vi "Get_OSC_DS1104Z.vi"(9 "Timeout (10000 ms)":u32=10000, 10 "Channel (0: Channel 1)":u16(ring) items=["Channel 1", "Channel 2", "Channel 3", "Channel 4"], 11 "VISA resource name":refnum<visa-resource-name>) -> (3 "Waveform Data":waveform(dbl)(graph))   [LabVIEW 2018]
panel:
  in  "t":i16=-25
  out "VISA resource name out":refnum<visa-resource-name>
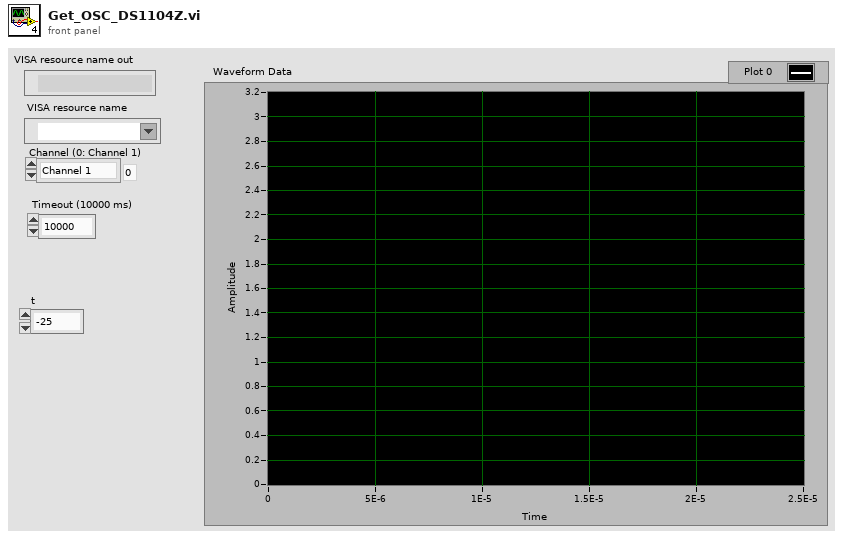
[diagram p1: front panel]
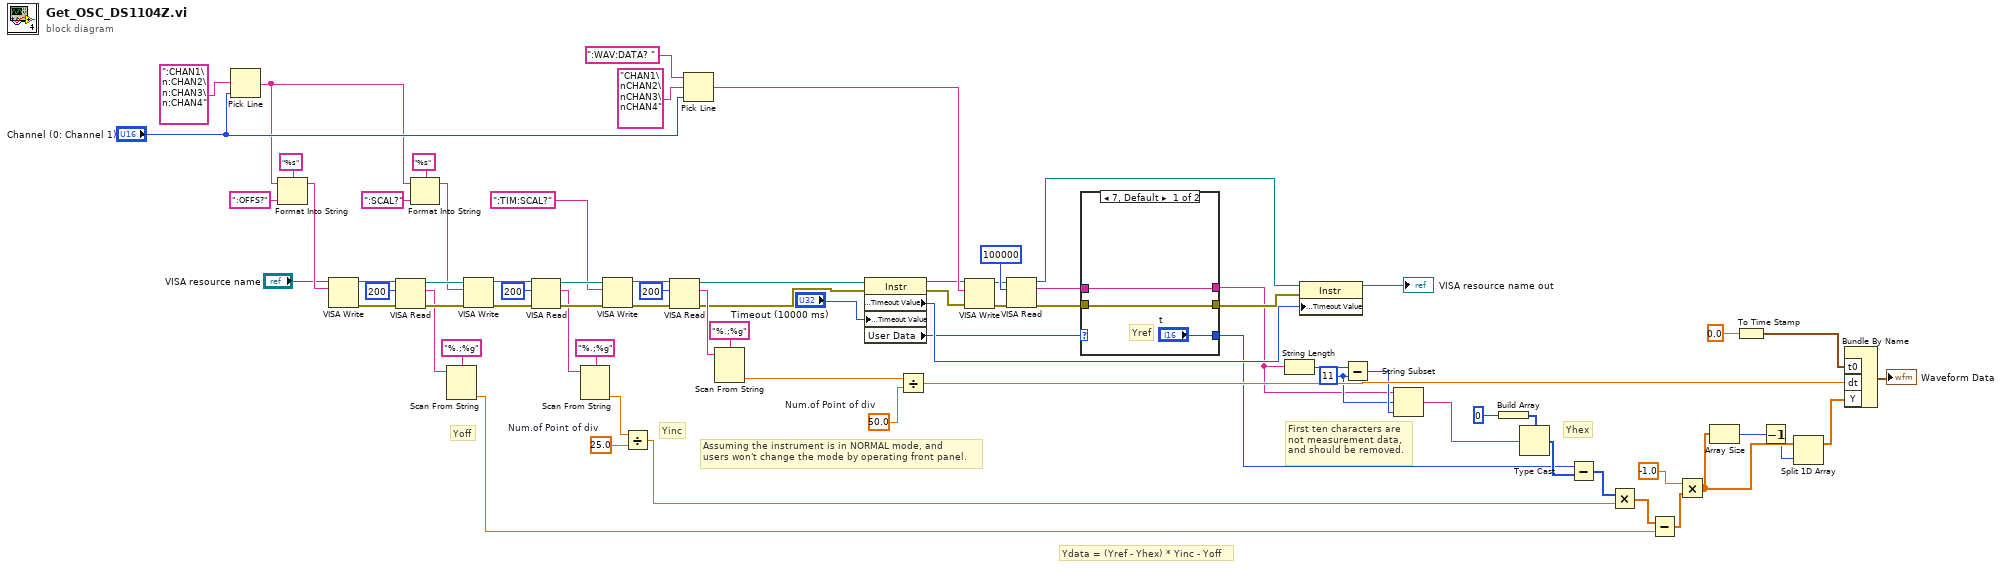
[diagram p0: block diagram]
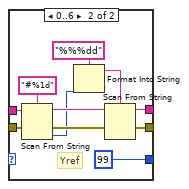
[diagram p2: hidden frame]
diagram:
  w14 = 11 ("y")
  w24 = 50.0  # Num.of Point of div
  w31 = 25.0  # Num.of Point of div
  # "Assuming the instrument is in NORMAL mode, and \nusers won't change the mode by operating front panel."
  # "First ten characters are\nnot measurement data, \nand should be removed."
  # "Yoff"
  # "Yinc"
  # "Yhex"
  # "Ydata = (Yref - Yhex) * Yinc - Yoff"
  n1 = Pick Line(multi-line string=":CHAN1\n:CHAN2\n:CHAN3\n:CHAN4" ("多行字符串"), line index="Channel (0: Channel 1)") -> (output string=w40:string)  [unwired: 1 out]
  n2 = Format Into String(format string="%s" ("格式字符串"), initial string=w40, ":OFFS?") -> (resulting string=w37:string)  [unwired: 1 in, 1 out]
  n3 = VISA Write(VISA resource name="VISA resource name", write buffer=w37) -> (VISA resource name out=w56:refnum<visa-resource-name>, error out=w55:errorcluster)  [unwired: 1 in, 1 out]
  n4 = VISA Read(VISA resource name=w56, byte count=u32 200, error in (no error)=w55) -> (VISA resource name out=w48:refnum<visa-resource-name>, read buffer=w39:string, error out=w47:errorcluster)  [unwired: 1 out]
  n5 = Format Into String(format string="%s" ("格式字符串"), initial string=w40, ":SCAL?") -> (resulting string=w36:string)  [unwired: 1 in, 1 out]
  n6 = Scan From String(format string="%.;%g", input string=w39) -> (output 1=w25:dbl)  [unwired: 2 in, 4 out]
  n7 = VISA Write(VISA resource name=w48, write buffer=w36, error in (no error)=w47) -> (VISA resource name out=w53:refnum<visa-resource-name>, error out=w54:errorcluster)  [unwired: 1 out]
  n8 = VISA Read(VISA resource name=w53, byte count=u32 200, error in (no error)=w54) -> (VISA resource name out=w44:refnum<visa-resource-name>, read buffer=w32:string, error out=w43:errorcluster)  [unwired: 1 out]
  n9 = Scan From String(format string="%.;%g", input string=w32) -> (output 1=w29:dbl)  [unwired: 2 in, 4 out]
  n10 = VISA Write(VISA resource name=w44, write buffer=":TIM:SCAL?", error in (no error)=w43) -> (VISA resource name out=w50:refnum<visa-resource-name>, error out=w49:errorcluster)  [unwired: 1 out]
  n11 = Divide(x=w29, y=w31) -> (x/y=w27:dbl)
  n12 = VISA Read(VISA resource name=w50, byte count=u32 200, error in (no error)=w49) -> (VISA resource name out=w3:refnum<visa-resource-name>, read buffer=w34:string, error out=w2:errorcluster)  [unwired: 1 out]
  n13 = Pick Line(string ("")=":WAV:DATA? " ("write buffer"), multi-line string="CHAN1\nCHAN2\nCHAN3\nCHAN4" ("多行字符串"), line index="Channel (0: Channel 1)") -> (output string=w59:string)
  n14 = Scan From String(format string="%.;%g", input string=w34) -> (output 1=w4:dbl)  [unwired: 2 in, 4 out]
  n15 = property class="Instr"(reference=w3, error in=w2, "General Settings:Timeout Value"="Timeout (10000 ms)") -> (reference out=w18:refnum<visa-resource-name>, error out=w20:errorcluster, "General Settings:Timeout Value"=w65:u32, "User Data"=w22:u32)
  n16 = Divide(x=w4, y=w24) -> (x/y=w23:dbl)
  n17 = VISA Write(VISA resource name=w18, write buffer=w59, error in (no error)=w20) -> (VISA resource name out=w17:refnum<visa-resource-name>, error out=w19:errorcluster)  [unwired: 1 out]
  n18 = VISA Read(VISA resource name=w17, byte count=u32 100000, error in (no error)=w19) -> (VISA resource name out=w68:refnum<visa-resource-name>, read buffer=w64:string, error out=w62:errorcluster)  [unwired: 1 out]
  n19 = case shown="7, Default" w22 {
    tunnel: [w78 w89] -> w13
    tunnel: [w77 w88] -> w67
    tunnel: w64 -> [w78 w81]
    tunnel: w62 -> [w77 w80]
    tunnel: ["t" i16 99 ("f")] -> w21
    frame 7, Default {
      # "Yref"
    }
    frame 0..6 {
      # "Yref"
      n20 = Scan From String(format string="#%1d", input string=w81, error in=w80) -> (remaining string=w85:string, error out=w83:errorcluster, output 1=w82:i32)  [unwired: 1 in, 2 out]
      n21 = Format Into String(format string="%%%dd", w82) -> (resulting string=w84:string)  [unwired: 2 in, 1 out]
      n22 = Scan From String(format string=w84, input string=w85, error in=w83) -> (remaining string=w89:string, error out=w88:errorcluster)  [unwired: 1 in, 3 out]
    }
  }
  n23 = String Length(string=w13) -> (length=w16:i32)
  n24 = property class="Instr"(reference=w68, error in=w67, "General Settings:Timeout Value"=w65) -> (reference out=→"VISA resource name out":refnum<visa-resource-name>)  [unwired: 1 out]
  n25 = Subtract(x=w16, y=w14) -> (x-y=w15:i32)
  n26 = String Subset(string=w13, offset (0)=w14, length (rest)=w15) -> (substring=w12:string)
  n27 = Build Array(u8 0) -> (w72:u8[])
  n28 = Type Cast(type=w72, x=w12) -> (*(type *) &x=w30:u8[])
  n29 = Subtract(x=w21, y=w30) -> (x-y=w28:i16[])
  n30 = Multiply(x=w28, y=w27) -> (x*y=w26:dbl[])
  n31 = Subtract(x=w26, y=w25) -> (x-y=w10:dbl[])
  n32 = Multiply(x=-1.0 ("x/y"), y=w10) -> (x*y=w8:dbl[])
  n33 = Array Size(array=w8) -> (size(s)=w5:i32)
  n34 = To Time Stamp(1:0.0 ("number")) -> (0:w73:timestamp)
  n35 = Decrement(x=w5) -> (x-1=w6:i32)
  n36 = Split 1D Array(array=w8, index=w6) -> (first subarray=w7:dbl[])  [unwired: 1 out]
  n37 = Bundle By Name("t0"=w73, "dt"=w23, "Y"=w7) -> (→"Waveform Data":waveform(dbl))  [unwired: 1 out]
